vi "Мультиплексор(4 5-разрядных операнда).vi"(0 "Inp0":T2, 1 "Inp1":T2, 2 "Inp2":T2, 3 "Inp3":T2, 4 "с":cluster{"с0":bool, "с1":bool}) -> (5 "r":T1)   [LabVIEW 2013]
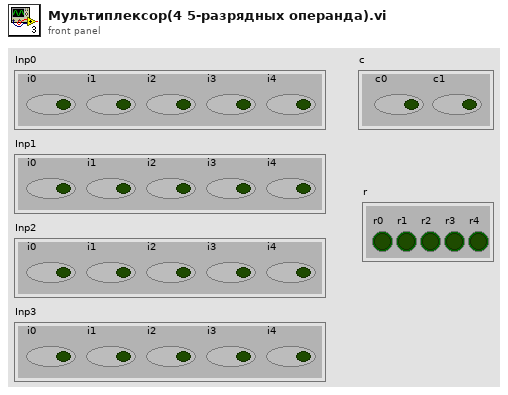
[diagram p1: front panel]
types:
  T1 = cluster{"r0":bool, "r1":bool, "r2":bool, "r3":bool, "r4":bool}
  T2 = cluster{"i0":bool, "i1":bool, "i2":bool, "i3":bool, "i4":bool}
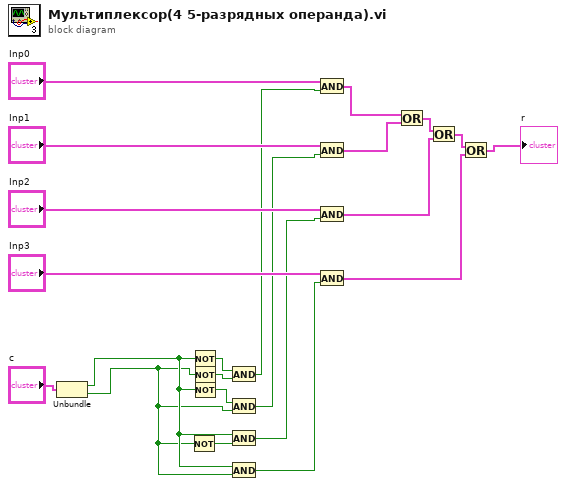
[diagram p0: block diagram]
diagram:
  n1 = Unbundle("с") -> ("с0"=w3:bool, "с1"=w1:bool)
  n2 = Not(x=w1) -> (.not. x?=w2:bool)
  n3 = Not(x=w3) -> (.not. x?=w17:bool)
  n4 = Not(x=w1) -> (.not. x?=w16:bool)
  n5 = Not(x=w3) -> (.not. x?=w4:bool)
  n6 = And(x=w17, y=w16) -> (x .and. y?=w15:bool)
  n7 = And(x=w4, y=w1) -> (x .and. y?=w14:bool)
  n8 = And(x=w3, y=w2) -> (x .and. y?=w13:bool)
  n9 = And(x=w3, y=w1) -> (x .and. y?=w12:bool)
  n10 = And(x="Inp0", y=w15) -> (x .and. y?=w11:T2)
  n11 = And(x="Inp1", y=w14) -> (x .and. y?=w10:T2)
  n12 = And(x="Inp2", y=w13) -> (x .and. y?=w8:T2)
  n13 = And(x="Inp3", y=w12) -> (x .and. y?=w6:T2)
  n14 = Or(x=w11, y=w10) -> (x .or. y?=w9:T2)
  n15 = Or(x=w9, y=w8) -> (x .or. y?=w7:T2)
  n16 = Or(x=w7, y=w6) -> (x .or. y?=→"r":T2)
